vi "Release.vi"(8 "error in (no error)":errorcluster, 11 "VacuumLine in":refnum<class "VacuumLine.lvclass">) -> (0 "error out":errorcluster, 3 "VacuumLine out":refnum<class "VacuumLine.lvclass">)   [LabVIEW 2016, in "Hardware.lvlib" / "VacuumLine.lvlib" / "VacuumLine.lvclass"]
uses:
  <userlib>/Common Components/Hardware/Abstract System/VacuumLine/VacuumLine/VacuumLine.lvclass
  <userlib>/Common Components/Hardware/Abstract System/VacuumLine/VacuumLine/VacuumLine.lvclass/VacuumLine.ctl
  <userlib>/Common Components/Hardware/LogicIO/LogicIO/LogicIO.lvclass
  <userlib>/Common Components/Hardware/Motor/Motor/Motor.lvclass
  <userlib>/Common Components/Hardware/Displacement Sensor/DispSnsr/DispSnsr.lvclass
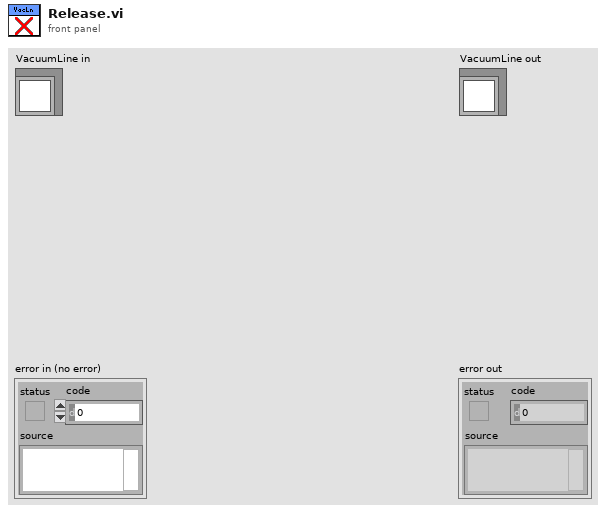
[diagram p1: front panel]
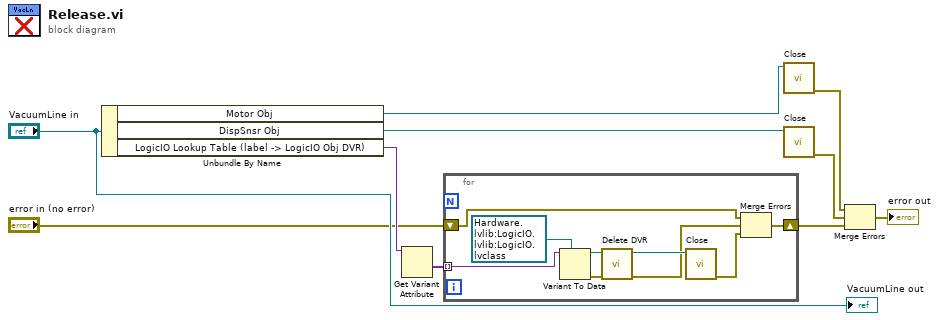
[diagram p0: block diagram]
diagram:
  n1 = Unbundle By Name("VacuumLine in") -> ("Motor Obj"=w2:refnum<class "Motor.lvclass">, "DispSnsr Obj"=w1:refnum<class "DispSnsr.lvclass">, "LogicIO Lookup Table (label -> LogicIO Obj DVR)"=w9:variant)
  n2 = Get Variant Attribute(Variant=w9) -> (values=w8:variant[])  [unwired: 3 in, 3 out]
  n3 = for {
    tunnel: w8 -> [w19] mode=indexing
    shift-right: [w18] -> w6
    shift-left: "error in (no error)" -> [w15]
    n4 = Variant To Data(type=refnum<data-value> refnum ("data value reference"), Variant=w19) -> (data=w16:refnum<data-value>, error out=w12:errorcluster)  [unwired: 1 in]
    n5 = call <userlib>:"Delete DVR.vi"("error in (no error)"=w12, "data value reference"=w16) -> ("error out"=w11:errorcluster, "LogicIO Obj"=w13:refnum<class "LogicIO.lvclass">)  [unwired: 8 in]
    n6 = call-dynamic "Close.vi"("LogicIO in"=w13) -> ("error out"=w17:errorcluster)  [unwired: 9 in, 1 out]
    n7 = Merge Errors(w15, w11, w17) -> (w18:errorcluster)
  }
  n8 = call-dynamic "Close.vi"("CCD in"=w2) -> ("error out"=w4:errorcluster)  [unwired: 9 in, 1 out]
  n9 = call-dynamic "Close.vi"("Displacement Sensor in"=w1) -> ("error out"=w3:errorcluster)  [unwired: 9 in, 1 out]
  n10 = Merge Errors(w4, w3, w6) -> (→"error out":errorcluster)
  "VacuumLine out" <- "VacuumLine in"
